vi "Data_Get Path.vi"(8 "error in (no error)":errorcluster, 11 "variant":variant) -> (0 "error out":errorcluster, 1 "Paths":variant, 3 "variant out":variant)   [LabVIEW 2015, in "Exposure Process.lvlib"]
uses:
  Exposure Process.lvlib
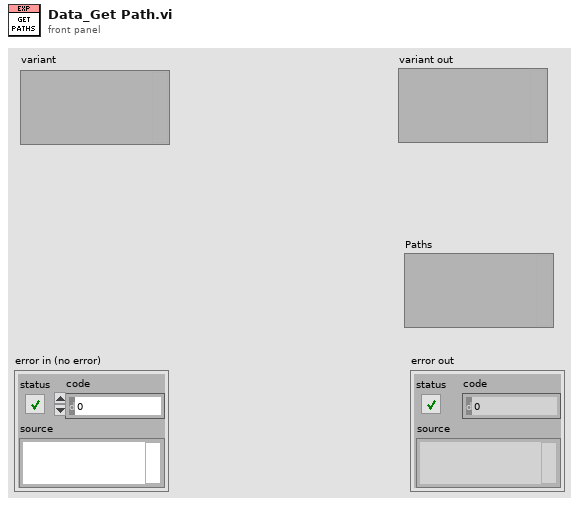
[diagram p1: front panel]
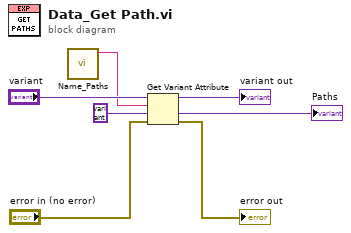
[diagram p0: block diagram]
diagram:
  n1 = call "Name_Paths.vi"() -> ("Name"=w4:string)  [unwired: 11 in]
  n2 = Get Variant Attribute(Variant="variant", name=w4, default value (empty Variant)=variant, error in="error in (no error)") -> (duplicate Variant=→"variant out":variant, value=→"Paths":variant, error out=→"error out":errorcluster)  [unwired: 1 out]
